vi "Measure DUT.vi"() -> (0 "error out":errorcluster, 2 "Boolean":bool, 3 "Array":dbl[][](array[numeric]))   [LabVIEW 2019]
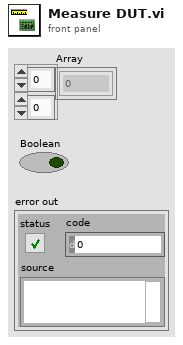
[diagram p1: front panel]
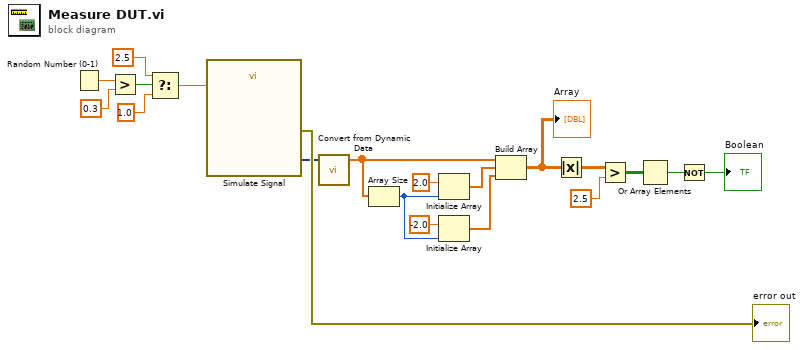
[diagram p0: block diagram]
diagram:
  n1 = Random Number (0-1)() -> (number: 0 to 1=w8:dbl)
  n2 = Greater?(x=w8, y=0.3) -> (0:w11:bool)
  n3 = Select(t=2.5 ("Amplitude"), s=w11, f=1.0) -> (s? t:f=w12:dbl)
  n4 = call "Simulate Signal"("Amplitude"=w12) -> ("Sine with Uniform Noise"=w1:dynamicdata, "error out"=→"error out":errorcluster)  [unwired: 13 in]
  n5 = call "Convert from Dynamic Data"("Dynamic Data Type"=w1) -> ("Array"=w2:dbl[])  [unwired: 3 in]
  n6 = Array Size(array=w2) -> (size(s)=w7:i32)
  n7 = Initialize Array(2.0 ("element"), w7) -> (w5:dbl[])
  n8 = Initialize Array(-2.0 ("element"), w7) -> (w6:dbl[])
  n9 = Build Array(w2, w5, w6) -> (w14:dbl[][])
  "Array" <- w14
  n10 = Absolute Value(x=w14) -> (abs(x)=w15:dbl[][])
  n11 = Greater?(x=w15, y=2.5 ("element")) -> (0:w17:bool[][])
  n12 = Or Array Elements(Boolean array=w17) -> (logical OR=w18:bool)
  n13 = Not(x=w18) -> (.not. x?=→"Boolean":bool)
